vi "DISP_WIND_TRAC_Y_SCAL_RPOS.vi"(0 "VISA IN":refnum<visa-resource-name>, 1 "Trace":i32, 2 "Position":i32, 5 "error in":errorcluster, 7 "Window":i32) -> (14 "VISA Out":refnum<visa-resource-name>, 19 "error out":errorcluster)   [LabVIEW 2018, in "PNA-X.lvlib"]
doc: "DISPlay:WINDow<wnum>:TRACe<tnum>:Y[:SCALe]:RPOSition <num> \n(Read-Write) Sets the Reference Position of the specified trace in the specified window \nParameters \n<wnum> Any existing window number. If unspecified, value is set to 1. \n<tnum> Any existing trace number; if unspecified, value is set to 1 \n<num> Reference position on the screen measured in horizontal graticules from the \nbottom. The range of acceptable values is dependent on format and domain. \nNote: This command will accept MIN or MAX instead of a numeric \nparameter. See SCPI Syntax for more information. \nExamples DISP:WIND:TRAC:Y:RPOS 0 \ndisplay:window2:trace2:y:rposition maximum \nQuery Syntax DISPlay:WINDow<wnum>:TRACe<tnum>:Y[:SCALe]:RPOSition? \nReturn Type Numeric \nDefault 5"
uses:
  PNA-X.lvlib
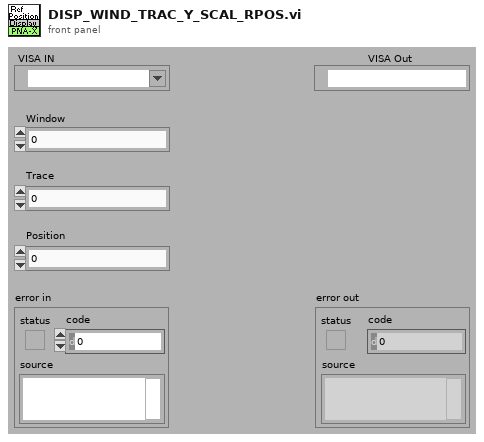
[diagram p1: front panel]
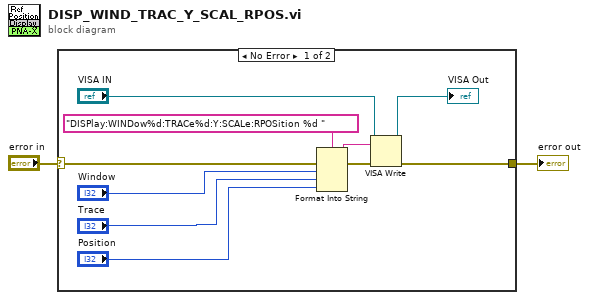
[diagram p0: block diagram]
diagram:
  n1 = case shown="No Error" "error in" {
    selector: "error in" -> [w12 w13]
    tunnel: [w7 w13] -> w1
    frame No Error {
      n2 = Format Into String(format string="DISPlay:WINDow%d:TRACe%d:Y:SCALe:RPOSition %d " ("Cmdline"), error in=w12, "Window", "Trace", "Position") -> (resulting string=w10:string, error out=w11:errorcluster)  [unwired: 1 in]
      n3 = VISA Write(VISA resource name="VISA IN", write buffer=w10, error in (no error)=w11) -> (VISA resource name out=→"VISA Out":refnum<visa-resource-name>, error out=w7:errorcluster)  [unwired: 1 out]
    }
    frame Error {
    }
  }
  "error out" <- w1
